vi "Server_ReadFile.vi"(8 "error in (no error)":errorcluster, 10 "Name":string="file.py", 11 "Server":path) -> (0 "error out":errorcluster, 2 "Code":string)   [LabVIEW 2020]
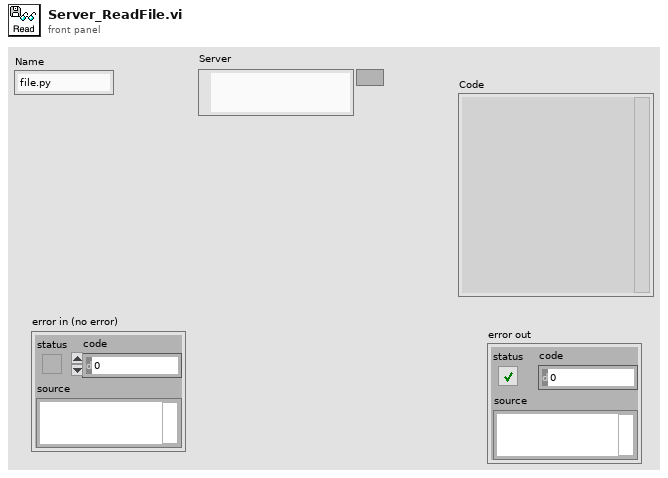
[diagram p1: front panel]
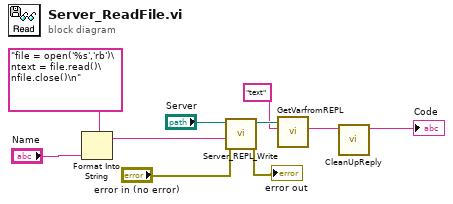
[diagram p0: block diagram]
diagram:
  n1 = Format Into String(format string="file = open('%s','rb')\ntext = file.read()\nfile.close()\n", "Name") -> (resulting string=w5:string)  [unwired: 2 in, 1 out]
  n2 = call "Server_REPL_Write.vi"("error in (no error)"="error in (no error)", "Code"=w5, "Server"="Server") -> ("error out"=→"error out":errorcluster)  [unwired: 8 in]
  n3 = call "GetVarfromREPL.vi"("Command"="text", "Server"="Server") -> ("reply"=w2:string)  [unwired: 8 in, 1 out]
  n4 = call "CleanUpReply.vi"("String"=w2) -> ("Cleaned string"=→"Code":string)  [unwired: 10 in]
